vi "Measurement.ReftoDVR.vi"(10 "Ref":u32 format="%08x") -> (2 "Ref":T1)   [LabVIEW 2017, in "Measurement.lvclass"]
doc: "JKI State Machine Objects (SMO) 1.0.0.5\nJKI - JKI\nCopyright (c) 2016, JKI"
uses:
  Measurement.lvclass
  Typedefs/PrivateData--Ref.ctl
  Typedefs/PrivateData--Cluster.ctl
  Typedefs/PublicEvents--Cluster.ctl
  Typedefs/PublicEvents--Measurement.Initialized.ctl
  Typedefs/Measurement.Measured--Data.ctl
  Typedefs/ProtectedEvents--Cluster.ctl
  Typedefs/ProtectedEvents--Measurement.Begin.ctl
  Typedefs/ProtectedEvents--Measurement.Pause.ctl
  Typedefs/ProtectedEvents--Measurement.End.ctl
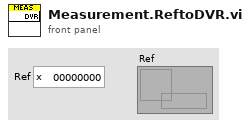
[diagram p1: front panel]
types:
  T1 = typedef "Measurement.lvclass/PrivateData--Ref.ctl" = refnum<data-value>
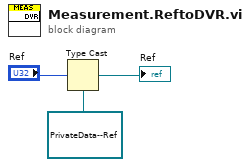
[diagram p0: block diagram]
diagram:
  n1 = Type Cast(type=T1 refnum ("Ref"), x="Ref") -> (*(type *) &x=→"Ref":T1)
